vi "Generate gRPC relevant name.vi"(11 "Project Name":string) -> (2 "gRPC proto File Name":string, 3 "gRPC Service Name":string)   [LabVIEW 2021, in "Plugin Generator.lvlib"]
uses:
  Plugin Generator.lvlib
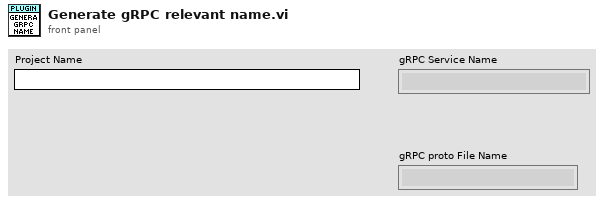
[diagram p1: front panel]
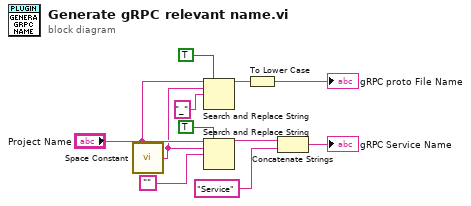
[diagram p0: block diagram]
diagram:
  n1 = call <vilib>:"Space Constant.vi"() -> ("String"=w6:string)
  n2 = Search and Replace String(replace all?=TRUE ("replace all? (F)"), input string="Project Name", search string=w6, replace string="_" ("replace string (\"\")")) -> (result string=w4:string)  [unwired: 4 in, 3 out]
  n3 = Search and Replace String(replace all?=TRUE ("replace all? (F)"), input string="Project Name", search string=w6, replace string="") -> (result string=w10:string)  [unwired: 4 in, 3 out]
  n4 = To Lower Case(string=w4) -> (all lower case string=→"gRPC proto File Name":string)
  n5 = Concatenate Strings(w10, "Service" ("string")) -> (→"gRPC Service Name":string)
